vi "set_user_defined_flag.vi"(4 "error in (no error)":errorcluster, 5 "Value":bool, 6 "Container State":T2, 7 "Display State In":T1) -> (0 "error out":errorcluster, 3 "Display State Out":T1)   [LabVIEW 2010, in "XSettings.xctl"]
uses:
  XSettings.xctl
  <vilib>/_xctls/Container State.ctl
  state.ctl
  <vilib>/_xctls/XControlSupport.lvlib
panel:
  # "Replace the Value Control below with a Control of desired type.\nDo not remove this Control or the others from the connector pane.\nDo not change the connector pane pattern.\nThe Value control should always be the third terminal from top on the input side in the connector pane."
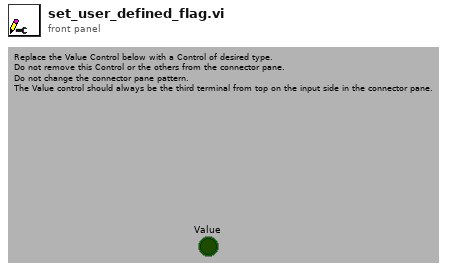
[diagram p1: front panel]
types:
  T1 = typedef "XSettings.xctl/state.ctl" = cluster{"error":errorcluster, "user-defined?":bool, "control refs":cluster{"settings combo":refnum<vi>}}
  T2 = typedef "XControlSupport.lvlib/Container State.ctl" = cluster{"Indicator?":bool, "Run Mode?":bool, " Refnum":refnum<vi>}
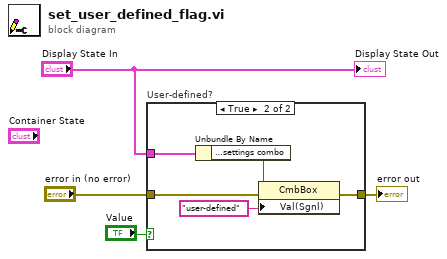
[diagram p0: block diagram]
diagram:
  n1 = case "User-defined?" shown="True" "Value" {
    tunnel: "error in (no error)" -> [w5 w8]
    tunnel: [w5 w7] -> w3
    tunnel: "Display State In" -> [_ w6]
    frame False {
    }
    frame True {
      n2 = Unbundle By Name(w6) -> ("control refs.settings combo"=w10:refnum<vi>)
      n3 = property class="CmbBox"(reference=w10, error in=w8, "Val(Sgnl)"="user-defined" ("Value (Signaling)")) -> (error out=w7:errorcluster)  [unwired: 1 out]
    }
  }
  "error out" <- w3
  "Display State Out" <- "Display State In"
